vi "Filter Source Node.vi"(7 "Supported Target Type":string="To Common Doc Dir", 8 "error in":errorcluster, 11 "Nodes Array in":refnum<k20>[](array[refnum])) -> (0 "error out":errorcluster, 3 "Nodes Array out":refnum<k20>[](array[refnum]))   [LabVIEW 2020, in "LVLIBP CD XML Updater.lvlib" / "Project XML Editor.lvclass"]
uses:
  Project XML Editor.lvclass
  <vilib>/xml/Close Reference(Node).vi
  <vilib>/xml/NI_XML.lvlib
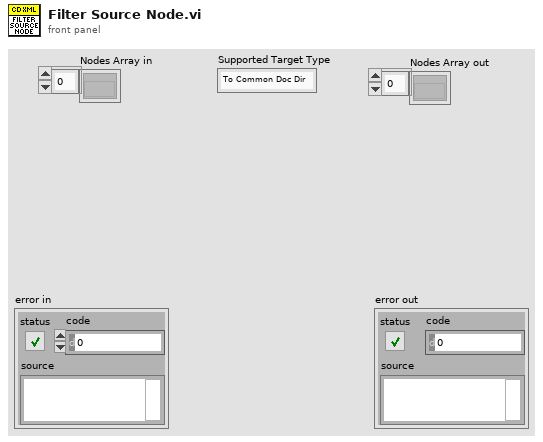
[diagram p1: front panel]
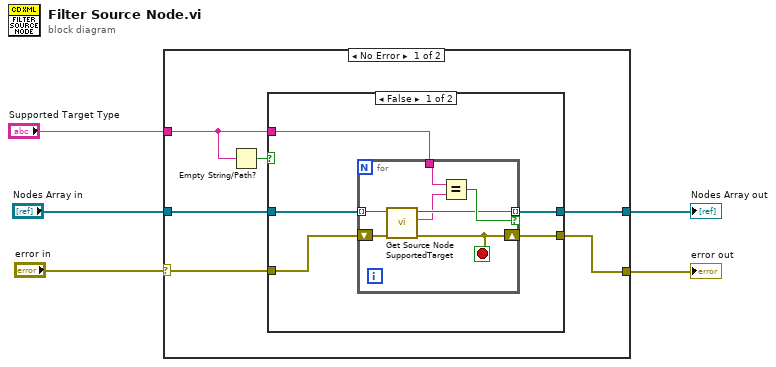
[diagram p0: block diagram]
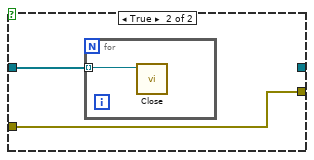
[diagram p2: hidden frame]
diagram:
  n1 = case shown="No Error" "error in" {
    selector: "error in" -> [w8 w27]
    tunnel: "Nodes Array in" -> [w11 w28]
    tunnel: [w10 w28] -> w4
    tunnel: [w9 w27] -> w3
    tunnel: "Supported Target Type" -> [w7 _]
    frame No Error {
      n2 = Empty String/Path?(string/path=w7) -> (empty?=w6:bool)
      n3 = case shown="False" w6 {
        tunnel: w11 -> [w16 w25]
        tunnel: [w15 _] -> w10
        tunnel: [w14 w24] -> w9
        tunnel: w8 -> [w13 w24]
        tunnel: w7 -> [w12 _]
        frame False {
          n4 = for {
            tunnel: [w19] -> w15 mode=indexing if=w23
            tunnel: w16 -> [w21] mode=indexing
            shift-right: [w18] -> w14
            shift-left: w13 -> [w20]
            tunnel: w12 -> [w22]
            stop <- w18 stop-if-true
            n5 = call "Get Source Node SupportedTarget.vi"("error in (no error)"=w20, "Node ref in"=w21) -> ("error out"=w18:errorcluster, "SupportedTarget out"=w17:string, "Node ref out"=w19:refnum<k20>)  [unwired: 6 in, 1 out]
            n6 = Equal?(x=w22, y=w17) -> (x = y?=w23:bool)
          }
        }
        frame True {
          n7 = for {
            tunnel: w25 -> [w26] mode=indexing
            n8 = call-poly <vilib>:"Close.vi"("node"=w26) -> ()  [unwired: 8 in, 1 out]
          }
        }
      }
    }
    frame Error {
    }
  }
  "Nodes Array out" <- w4
  "error out" <- w3
